vi "Total Energy Used.vi"(8 "Error In":errorcluster, 11 "110-130 Array":dbl[][](array[numeric])) -> (0 "Error Out":errorcluster, 2 "No Data Found Between 110-130":bool, 3 "Total Energy Expended (W-hr)":dbl)   [LabVIEW 2016]
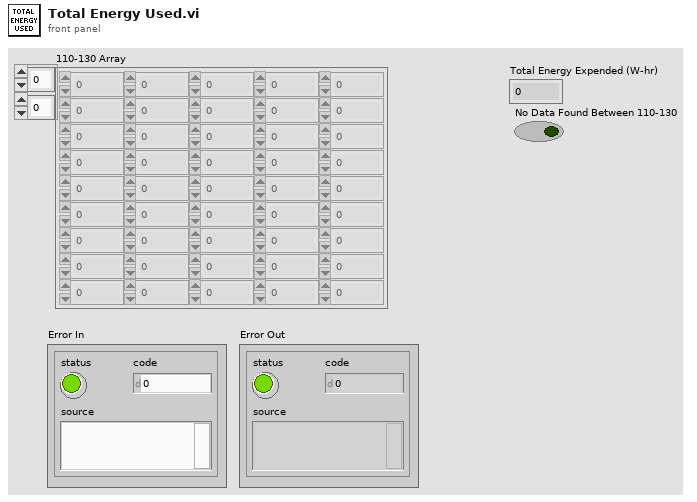
[diagram p1: front panel]
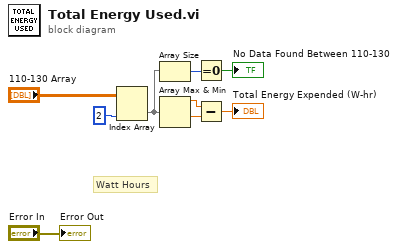
[diagram p0: block diagram]
diagram:
  # "Watt Hours"
  n1 = Index Array(array="110-130 Array", index (col)=2 ("disabled index (col)")) -> (element=w5:dbl[])  [unwired: 1 in]
  n2 = Array Size(array=w5) -> (size(s)=w6:i32)
  n3 = Array Max & Min(array=w5) -> (max value=w3:dbl, min value=w4:dbl)  [unwired: 2 out]
  n4 = Equal To 0?(x=w6) -> (x = 0?=→"No Data Found Between 110-130":bool)
  n5 = Subtract(x=w3, y=w4) -> (x-y=→"Total Energy Expended (W-hr)":dbl)
  "Error Out" <- "Error In"
